vi "Terminate.vi"(8 "error in (no error)":errorcluster, 10 "Message in":refnum<class "TerminateMessage.lvclass">, 11 "BMC in":refnum<class "BMC.lvclass">) -> (0 "error out":errorcluster, 3 "BMC out":refnum<class "BMC.lvclass">)   [LabVIEW 2012, in "BMC.lvclass"]
doc: "This member function is called when the statemachine in the run.vi receives an 'terminate' command. It closes the RabbitMQ connection. \n\nOverride this member function in your derived class to release all previously acquired resources (but don't forget to call the parent method). If your component has subcomponents, they count as resources, and you have to release them by calling their own terminate functions."
uses:
  BMC.lvclass
  <vilib>/Distrio/Murmex/TerminateMessage/TerminateMessage.lvclass
  <vilib>/Distrio/Murmex/Murmex/Murmex.lvclass
panel:
  # "This method is called when the TERMINATE\ntrigger is sent. \n\nOverride this method when your component needs to\nrespond to this trigger. \n\nCall parent for proper implementation"
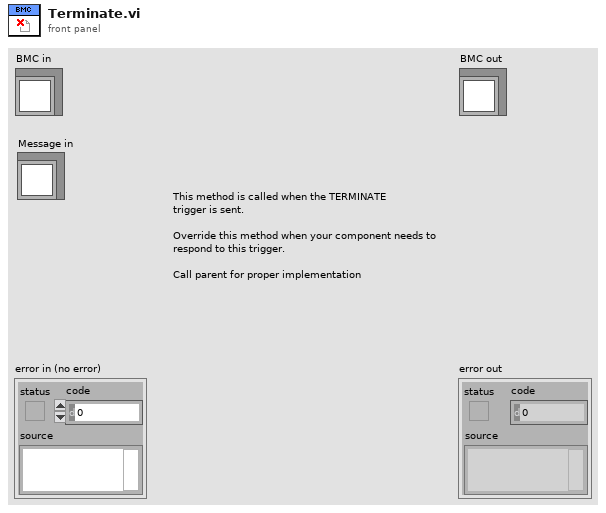
[diagram p1: front panel]
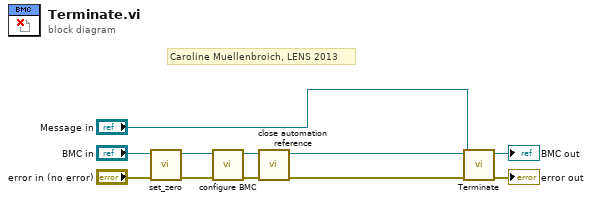
[diagram p0: block diagram]
diagram:
  # "Caroline Muellenbroich, LENS 2013"
  n1 = call-dynamic "set_zero.vi"("error in (no error)"="error in (no error)", "BMC in"="BMC in") -> ("error out"=w7:errorcluster, "BMC out"=w8:refnum<class "BMC.lvclass">)  [unwired: 8 in]
  n2 = call-dynamic "configure BMC.vi"("error in (no error)"=w7, "BMC in"=w8) -> ("error out"=w6:errorcluster, "BMC out"=w5:refnum<class "BMC.lvclass">)  [unwired: 8 in]
  n3 = call-dynamic "close automation reference.vi"("error in (no error)"=w6, "BMC in"=w5) -> ("error out"=w1:errorcluster, "BMC out"=w2:refnum<class "BMC.lvclass">)  [unwired: 8 in]
  n4 = call-parent "Terminate.vi"("error in (no error)"=w1, "Message in"="Message in", "Murmex in"=w2) -> ("error out"=→"error out":errorcluster, "Murmex out"=→"BMC out":refnum<class "BMC.lvclass">)  [unwired: 7 in]
